vi "Get Control Ref v1.vi"(8 "Control Name":string="General Tab", 11 "Controls Array":refnum<vi>[](array[refnum])) -> (3 "Ctl Refnum Out":refnum<vi>)   [LabVIEW 2014]
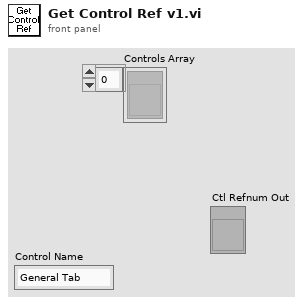
[diagram p1: front panel]
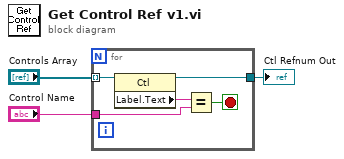
[diagram p0: block diagram]
diagram:
  n1 = for {
    tunnel: "Controls Array" -> [w6] mode=indexing
    tunnel: [w5] -> w1
    tunnel: "Control Name" -> [w4]
    stop <- w7 stop-if-true
    n2 = property class="Ctl"(reference=w6) -> (reference out=w5:refnum<vi>, "Label.Text"=w8:string)  [unwired: 1 in, 1 out]
    n3 = Equal?(x=w8, y=w4) -> (x = y?=w7:bool)
  }
  "Ctl Refnum Out" <- w1
